vi "set_rotation.vi"(8 "error in (no error)":errorcluster, 9 "x angle (rotation angle, phi)":dbl[unit], 10 "z angle (rotation angle, phi)":dbl[unit], 11 "FPGAWrapperMH120124FrameScan_PXI7813R in":refnum<class "FPGAWrapperMH120124FrameScan_PXI7813R.lvclass">) -> (0 "error out":errorcluster, 3 "FPGAWrapperMH120124FrameScan_PXI7813R out":refnum<class "FPGAWrapperMH120124FrameScan_PXI7813R.lvclass">)   [LabVIEW 2010, in "FPGAWrapperMH120124FrameScan_PXI7813R.lvclass"]
uses:
  FPGAWrapperMH120124FrameScan_PXI7813R.lvclass
  FPGAWrapperMH120124FrameScan_PXI7813R.lvclass/FPGAWrapperMH120124FrameScan_PXI7813R.ctl
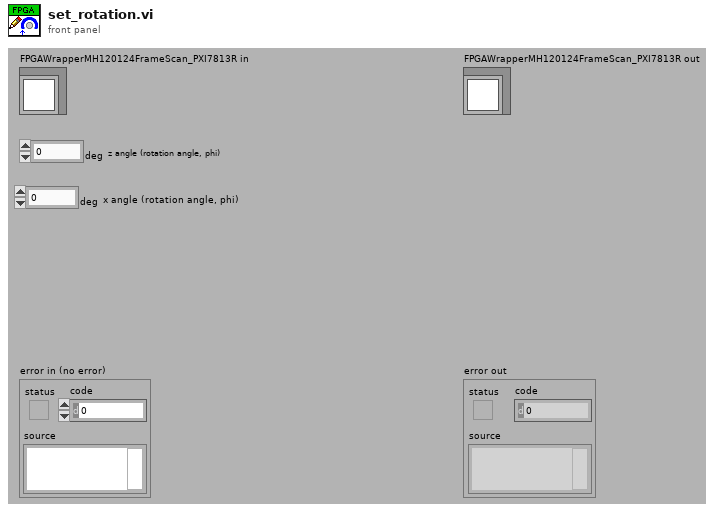
[diagram p1: front panel]
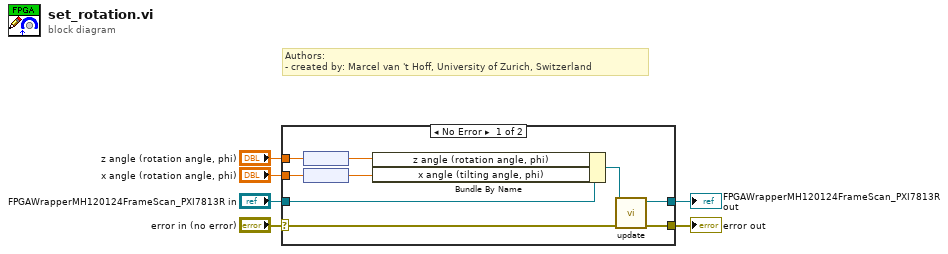
[diagram p0: block diagram]
diagram:
  # "Authors: \n- created by: Marcel van 't Hoff, University of Zurich, Switzerland"
  n1 = case shown="No Error" "error in (no error)" {
    selector: "error in (no error)" -> [w8 w16]
    tunnel: [w7 w16] -> w5
    tunnel: [w9 w17] -> w3
    tunnel: "FPGAWrapperMH120124FrameScan_PXI7813R in" -> [w15 w17]
    tunnel: "z angle (rotation angle, phi)" -> [w14 _]
    tunnel: "x angle (rotation angle, phi)" -> [w11 _]
    frame No Error {
      n2 = node(w14) -> (w13:dbl)
      n3 = node(w11) -> (w12:dbl)
      n4 = Bundle By Name(cluster=w15, "z angle (rotation angle, phi)"=w13, "x angle (tilting angle, phi)"=w12) -> (w10:refnum<class "FPGAWrapperMH120124FrameScan_PXI7813R.lvclass">)
      n5 = call-dynamic "update.vi"("error in (no error)"=w8, "FPGAWrapperMH120124FrameScan_PXI7813R in"=w10) -> ("error out"=w7:errorcluster, "FPGAWrapperMH120124FrameScan_PXI7813R out"=w9:refnum<class "FPGAWrapperMH120124FrameScan_PXI7813R.lvclass">)  [unwired: 8 in]
    }
    frame Error {
    }
  }
  "error out" <- w5
  "FPGAWrapperMH120124FrameScan_PXI7813R out" <- w3
